vi "MDrive_Set_Parameter.vi"(4 "error out 2":errorcluster, 5 "Parameter Setpoint":string, 6 "Set Parameter":T1, 7 "VISA resource name out 2":refnum<visa-resource-name>) -> (0 "error out":errorcluster, 1 "read buffer":string, 3 "VISA resource name out":refnum<visa-resource-name>)   [LabVIEW 2013]
uses:
  Set Parameter.ctl
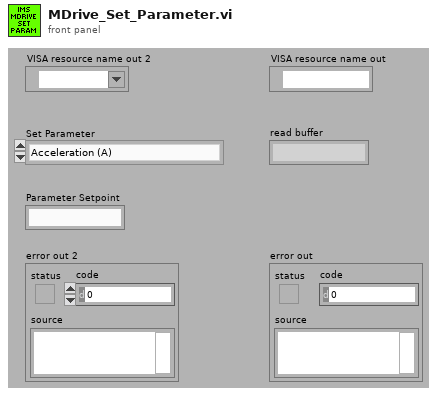
[diagram p1: front panel]
types:
  T1 = typedef "Set Parameter.ctl" = enum16{"Acceleration (A)", "Baud Rate (BD)", "Counter 1 (C1)", "Counter 2 (C2)", "Control C Software Reset (CE)", "Check Sum Enable (CK)", "Clock Mode (CM)", "Clock Mode Ratio (CR)", "Clock Mode Out Step Width (CW)", "Deceleration (D)", "Digital Filtering, Input 1 (D1)", "Digital Filtering, Input 2 (D2)", "Digital Filtering, Input 3 (D3)", "Digital Filtering, Input 4 (D4)", "Digital Filtering, Input 5 (D5)", "Digital Filtering, Input 9 (D9)", "Digital Filtering, Input 10 (D10)", "Digital Filtering, Input 11 (D11)", "Digital Filtering, Input 12 (D12)", "Deadband (DB)", "Decrement Variable (DC)", "Enable/Disable Drive (DE)", "Device Name (DN)", "End Program Execution (E)", "Encoder Function Enable (EE)", "Encoder Lines (EL)", "Echo Mode (EM)", "Escape (ES)", "Execute Program at Address (EX)", "Hold (H)", "Hold Current (HC)", "Hold Current Delay Time (HI)", "Home to Encoder Index (HM)", "Home to Home Switch (HT)", "Increment Variable (IC)", "Initialize Parameters to NVM (IP)", "Input into Variable (IV)", "Jog Enable (JE)", "Limit Stop Mode (LM)", "Move Absolute (MA)", "Move Relative (MR)", "MicroStepping Select (MS)", "Motor Settling Delay Time (MT)", "Output 1 (O1)", "Output 2 (O2)", "Output 3 (O3)", "Output 4 (O4)", "Output 9 (O9)", "Output 10 (O10)", "Output 11 (O11)", "Output 12 (O12)", "Output High Byte (9-12) (OH)", "Output Low Byte (1-4) (OL)", "Output Total (1-4 and 9-12) (OT)", "Position Maintenance (PM)", "Party Mode (PY)", "Register 1 (R1)", "Register 2 (R2)", "Register 3 (R3)", "Register 4 (R4)", "Run Current (RC)", "Stall Factor (SF)", "Slew (SL)", "Stall Mode Set (SM)", "Upgrade Firmware (UG)", "Velocity Initial (VI)", "Velocity Maximum (VM)"}
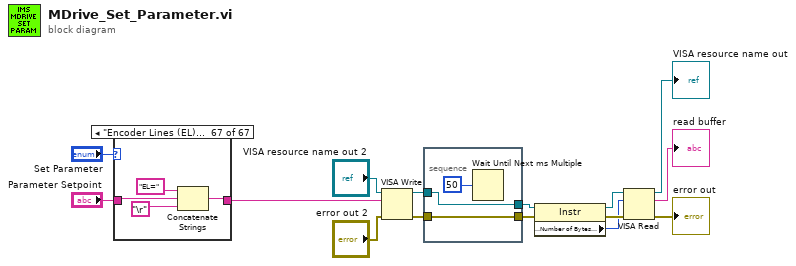
[diagram p0: block diagram]
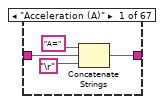
[diagram p2: hidden frame]
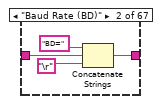
[diagram p3: hidden frame]
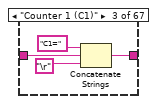
[diagram p4: hidden frame]
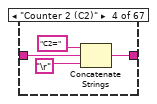
[diagram p5: hidden frame]
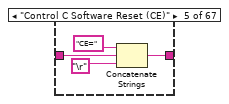
[diagram p6: hidden frame]
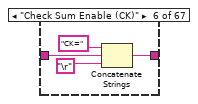
[diagram p7: hidden frame]
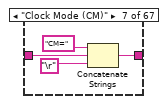
[diagram p8: hidden frame]
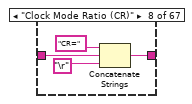
[diagram p9: hidden frame]
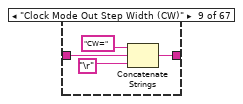
[diagram p10: hidden frame]
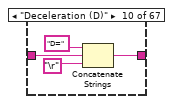
[diagram p11: hidden frame]
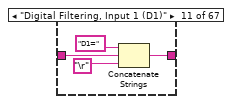
[diagram p12: hidden frame]
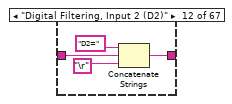
[diagram p13: hidden frame]
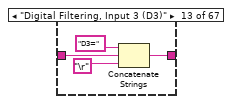
[diagram p14: hidden frame]
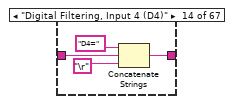
[diagram p15: hidden frame]
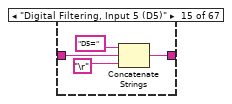
[diagram p16: hidden frame]
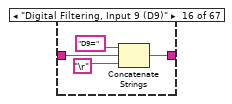
[diagram p17: hidden frame]
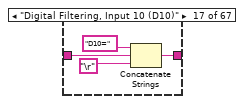
[diagram p18: hidden frame]
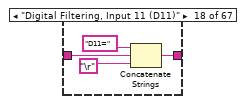
[diagram p19: hidden frame]
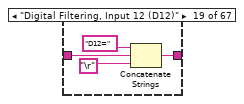
[diagram p20: hidden frame]
diagram:
  n1 = case shown="\"Encoder Lines (EL)\"" "Set Parameter" {
    tunnel: "Parameter Setpoint" -> [w17 w20 w25 w29 w32 w36 w40 w44 w48 w52 w56 w60 w64 w68 w72 w76 w80 w84 w88 w92 w96 w100 w104 w108 w112 w116 w120 w124 w128 w132 w136 w140 w144 w148 w152 w156 w160 w164 w168 w172 w176 w180 w184 w188 w192 w196 w200 w204 w208 w212 w216 w220 w224 w228 w232 w237 w240 w244 w248 w252 w256 w260 w264 w268 w272 w277 w280]
    tunnel: [w16 w21 w24 w28 w33 w37 w41 w45 w49 w53 w57 w61 w65 w69 w73 w77 w81 w85 w89 w93 w97 w101 w105 w109 w113 w117 w121 w125 w129 w133 w137 w141 w145 w149 w153 w157 w161 w165 w169 w173 w177 w181 w185 w189 w193 w197 w201 w205 w209 w213 w217 w221 w225 w229 w233 w236 w241 w245 w249 w253 w257 w261 w265 w269 w273 w276 w281] -> w1
    frame "Acceleration (A)" {
      n2 = Concatenate Strings("A=" ("string"), w17, "\r") -> (w16:string)
    }
    frame "Baud Rate (BD)" {
      n3 = Concatenate Strings("BD=" ("string"), w20, "\r") -> (w21:string)
    }
    frame "Counter 1 (C1)" {
      n4 = Concatenate Strings("C1=" ("string"), w25, "\r") -> (w24:string)
    }
    frame "Counter 2 (C2)" {
      n5 = Concatenate Strings("C2=" ("string"), w29, "\r") -> (w28:string)
    }
    frame "Control C Software Reset (CE)" {
      n6 = Concatenate Strings("CE=" ("string"), w32, "\r") -> (w33:string)
    }
    frame "Check Sum Enable (CK)" {
      n7 = Concatenate Strings("CK=" ("string"), w36, "\r") -> (w37:string)
    }
    frame "Clock Mode (CM)" {
      n8 = Concatenate Strings("CM=" ("string"), w40, "\r") -> (w41:string)
    }
    frame "Clock Mode Ratio (CR)" {
      n9 = Concatenate Strings("CR=" ("string"), w44, "\r") -> (w45:string)
    }
    frame "Clock Mode Out Step Width (CW)" {
      n10 = Concatenate Strings("CW=" ("string"), w48, "\r") -> (w49:string)
    }
    frame "Deceleration (D)" {
      n11 = Concatenate Strings("D=" ("string"), w52, "\r") -> (w53:string)
    }
    frame "Digital Filtering, Input 1 (D1)" {
      n12 = Concatenate Strings("D1=" ("string"), w56, "\r") -> (w57:string)
    }
    frame "Digital Filtering, Input 2 (D2)" {
      n13 = Concatenate Strings("D2=" ("string"), w60, "\r") -> (w61:string)
    }
    frame "Digital Filtering, Input 3 (D3)" {
      n14 = Concatenate Strings("D3=" ("string"), w64, "\r") -> (w65:string)
    }
    frame "Digital Filtering, Input 4 (D4)" {
      n15 = Concatenate Strings("D4=" ("string"), w68, "\r") -> (w69:string)
    }
    frame "Digital Filtering, Input 5 (D5)" {
      n16 = Concatenate Strings("D5=" ("string"), w72, "\r") -> (w73:string)
    }
    frame "Digital Filtering, Input 9 (D9)" {
      n17 = Concatenate Strings("D9=" ("string"), w76, "\r") -> (w77:string)
    }
    frame "Digital Filtering, Input 10 (D10)" {
      n18 = Concatenate Strings("D10=" ("string"), w80, "\r") -> (w81:string)
    }
    frame "Digital Filtering, Input 11 (D11)" {
      n19 = Concatenate Strings("D11=" ("string"), w84, "\r") -> (w85:string)
    }
    frame "Digital Filtering, Input 12 (D12)" {
      n20 = Concatenate Strings("D12=" ("string"), w88, "\r") -> (w89:string)
    }
    frame "Deadband (DB)" {
      n21 = Concatenate Strings("DB=" ("string"), w92, "\r") -> (w93:string)
    }
    frame "Decrement Variable (DC)" {
      n22 = Concatenate Strings("DC=" ("string"), w96, "\r") -> (w97:string)
    }
    frame "Enable/Disable Drive (DE)" {
      n23 = Concatenate Strings("DE=" ("string"), w100, "\r") -> (w101:string)
    }
    frame "Device Name (DN)" {
      n24 = Concatenate Strings("DN=" ("string"), w104, "\r") -> (w105:string)
    }
    frame "End Program Execution (E)" {
      n25 = Concatenate Strings("E=" ("string"), w108, "\r") -> (w109:string)
    }
    frame "Encoder Function Enable (EE)" {
      n26 = Concatenate Strings("EE=" ("string"), w112, "\r") -> (w113:string)
    }
    frame "Echo Mode (EM)" {
      n27 = Concatenate Strings("EM=" ("string"), w116, "\r") -> (w117:string)
    }
    frame "Escape (ES)" {
      n28 = Concatenate Strings("ES=" ("string"), w120, "\r") -> (w121:string)
    }
    frame "Execute Program at Address (EX)" {
      n29 = Concatenate Strings("EX=" ("string"), w124, "\r") -> (w125:string)
    }
    frame "Hold (H)" {
      n30 = Concatenate Strings("H=" ("string"), w128, "\r") -> (w129:string)
    }
    frame "Hold Current (HC)" {
      n31 = Concatenate Strings("HC=" ("string"), w132, "\r") -> (w133:string)
    }
    frame "Hold Current Delay Time (HI)" {
      n32 = Concatenate Strings("HI=" ("string"), w136, "\r") -> (w137:string)
    }
    frame "Home to Encoder Index (HM)" {
      n33 = Concatenate Strings("HM=" ("string"), w140, "\r") -> (w141:string)
    }
    frame "Home to Home Switch (HT)" {
      n34 = Concatenate Strings("HT=" ("string"), w144, "\r") -> (w145:string)
    }
    frame "Increment Variable (IC)" {
      n35 = Concatenate Strings("IC=" ("string"), w148, "\r") -> (w149:string)
    }
    frame "Initialize Parameters to NVM (IP)" {
      n36 = Concatenate Strings("IP=" ("string"), w152, "\r") -> (w153:string)
    }
    frame "Input into Variable (IV)" {
      n37 = Concatenate Strings("IV=" ("string"), w156, "\r") -> (w157:string)
    }
    frame "Jog Enable (JE)" {
      n38 = Concatenate Strings("JE=" ("string"), w160, "\r") -> (w161:string)
    }
    frame "Limit Stop Mode (LM)" {
      n39 = Concatenate Strings("LM=" ("string"), w164, "\r") -> (w165:string)
    }
    frame "Move Absolute (MA)" {
      n40 = Concatenate Strings("MA=" ("string"), w168, "\r") -> (w169:string)
    }
    frame "Move Relative (MR)" {
      n41 = Concatenate Strings("MR=" ("string"), w172, "\r") -> (w173:string)
    }
    frame "MicroStepping Select (MS)" {
      n42 = Concatenate Strings("MS=" ("string"), w176, "\r") -> (w177:string)
    }
    frame "Motor Settling Delay Time (MT)" {
      n43 = Concatenate Strings("MT=" ("string"), w180, "\r") -> (w181:string)
    }
    frame "Output 1 (O1)" {
      n44 = Concatenate Strings("O1=" ("string"), w184, "\r") -> (w185:string)
    }
    frame "Output 2 (O2)" {
      n45 = Concatenate Strings("O2=" ("string"), w188, "\r") -> (w189:string)
    }
    frame "Output 3 (O3)" {
      n46 = Concatenate Strings("O3=" ("string"), w192, "\r") -> (w193:string)
    }
    frame "Output 4 (O4)" {
      n47 = Concatenate Strings("O4=" ("string"), w196, "\r") -> (w197:string)
    }
    frame "Output 9 (O9)" {
      n48 = Concatenate Strings("O9=" ("string"), w200, "\r") -> (w201:string)
    }
    frame "Output 10 (O10)" {
      n49 = Concatenate Strings("O10=" ("string"), w204, "\r") -> (w205:string)
    }
    frame "Output 11 (O11)" {
      n50 = Concatenate Strings("O11=" ("string"), w208, "\r") -> (w209:string)
    }
    frame "Output 12 (O12)" {
      n51 = Concatenate Strings("O12=" ("string"), w212, "\r") -> (w213:string)
    }
    frame "Output High Byte (9-12) (OH)" {
      n52 = Concatenate Strings("OH=" ("string"), w216, "\r") -> (w217:string)
    }
    frame "Output Low Byte (1-4) (OL)" {
      n53 = Concatenate Strings("OL=" ("string"), w220, "\r") -> (w221:string)
    }
    frame "Output Total (1-4 and 9-12) (OT)" {
      n54 = Concatenate Strings("OT=" ("string"), w224, "\r") -> (w225:string)
    }
    frame "Position Maintenance (PM)" {
      n55 = Concatenate Strings("PM=" ("string"), w228, "\r") -> (w229:string)
    }
    frame "Party Mode (PY)" {
      n56 = Concatenate Strings("PY=" ("string"), w232, "\r") -> (w233:string)
    }
    frame "Register 1 (R1)" {
      n57 = Concatenate Strings("R1=" ("string"), w237, "\r") -> (w236:string)
    }
    frame "Register 2 (R2)" {
      n58 = Concatenate Strings("R2=" ("string"), w240, "\r") -> (w241:string)
    }
    frame "Register 3 (R3)" {
      n59 = Concatenate Strings("R3=" ("string"), w244, "\r") -> (w245:string)
    }
    frame "Register 4 (R4)" {
      n60 = Concatenate Strings("R4=" ("string"), w248, "\r") -> (w249:string)
    }
    frame "Run Current (RC)" {
      n61 = Concatenate Strings("RC=" ("string"), w252, "\r") -> (w253:string)
    }
    frame "Stall Factor (SF)" {
      n62 = Concatenate Strings("SF=" ("string"), w256, "\r") -> (w257:string)
    }
    frame "Slew (SL)" {
      n63 = Concatenate Strings("SL=" ("string"), w260, "\r") -> (w261:string)
    }
    frame "Stall Mode Set (SM)" {
      n64 = Concatenate Strings("SM=" ("string"), w264, "\r") -> (w265:string)
    }
    frame "Upgrade Firmware (UG)" {
      n65 = Concatenate Strings("UG=" ("string"), w268, "\r") -> (w269:string)
    }
    frame "Velocity Initial (VI)" {
      n66 = Concatenate Strings("VI=" ("string"), w272, "\r") -> (w273:string)
    }
    frame "Velocity Maximum (VM)" {
      n67 = Concatenate Strings("VM=" ("string"), w277, "\r") -> (w276:string)
    }
    frame "Encoder Lines (EL)" {
      n68 = Concatenate Strings("EL=" ("string"), w280, "\r") -> (w281:string)
    }
  }
  n69 = VISA Write(VISA resource name="VISA resource name out 2", write buffer=w1, error in (no error)="error out 2") -> (VISA resource name out=w7:refnum<visa-resource-name>, error out=w6:errorcluster)  [unwired: 1 out]
  n70 = stacked-sequence {
    tunnel: w7 -> [w286]
    tunnel: w6 -> [w285]
    tunnel: [w286] -> w5
    tunnel: [w285] -> w4
    frame #0 {
      n71 = Wait Until Next ms Multiple(millisecond multiple=u32 50) -> ()  [unwired: 1 out]
    }
  }
  n72 = property class="Instr"(reference=w5, error in=w4) -> (reference out=w13:refnum<visa-resource-name>, error out=w12:errorcluster, "Serial Settings:Number of Bytes at Serial Port"=w11:u32)
  n73 = VISA Read(VISA resource name=w13, byte count=w11, error in (no error)=w12) -> (VISA resource name out=→"VISA resource name out":refnum<visa-resource-name>, read buffer=→"read buffer":string, error out=→"error out":errorcluster)  [unwired: 1 out]
